vi "ReadMessage.vi"(0 "reference":refnum<class "VdTcpIP.lvclass">, 2 "MaxBytesToRead(10000)":u32=10000, 3 "Binary":bool, 4 "timeout ms (25000)":i32=25000, 5 "error in (no error)":errorcluster, 6 "mode (standard)":T1(ring)) -> (14 "reference out":refnum<class "VdTcpIP.lvclass">, 15 "Message":string, 19 "error out":errorcluster)   [LabVIEW 2020, in "VdTcpIP.lvclass"]
doc: "Reads a message"
uses:
  VdTcpIP.lvclass
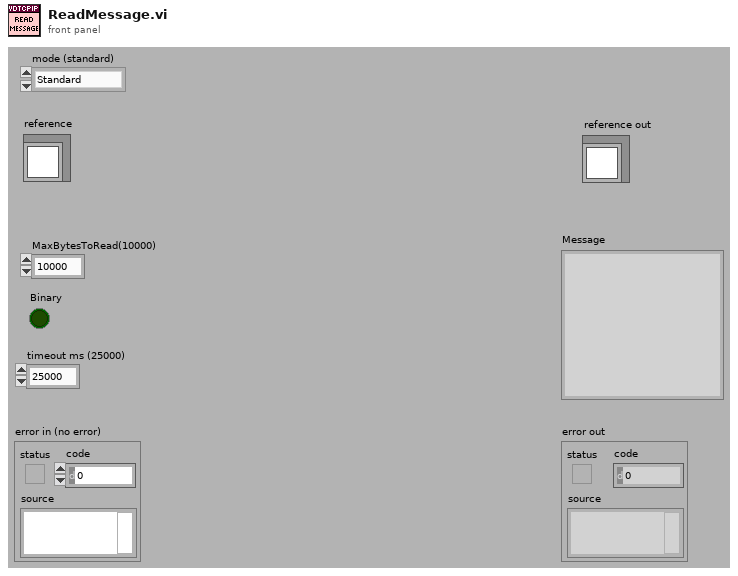
[diagram p1: front panel]
types:
  T1 = enum16{"Standard", "Buffered", "CRLF", "Immediate"}
  T2 = typedef "VdTcpIP.lvclass/ObjectAttributes.ctl" = cluster{"IP-Address":string, "Port":u16, "Connection":refnum<k5>, "Listener":refnum<k5>, "ListenerConnection":refnum<k5>, "Listner":bool, "ListnerProcessRunning":bool, "InConnections":refnum<k5>[], "InConnectionsIP":string[], "InConnectionAdded":refnum<notifier>, "RunVIOnNewConnection":variant, "DataToNewConnectionVI":cluster{"ControlName":string, "ControlValue":variant}[], "WebServicesURL_Location(http://...)":string, "WebServicesPostWebPage(*.asmx)":string, "Semaphore":T3, "AutoReConnectTimes":i32, "AutoReConnectInterval(ms)":i32, "ConnectionTimeout":i32}
  T3 = typedef "Semaphore RefNum" = refnum<k1>
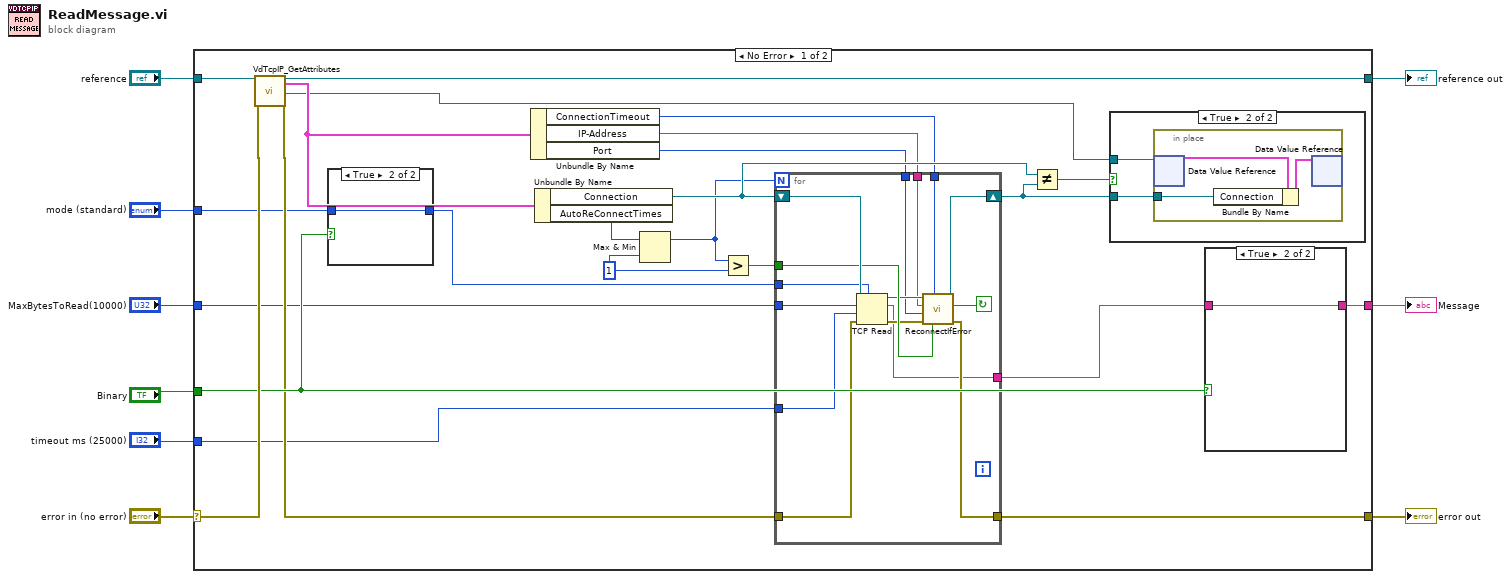
[diagram p0: block diagram]
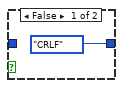
[diagram p3: hidden frame]
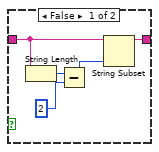
[diagram p4: hidden frame]
diagram:
  n1 = case shown="No Error" "error in (no error)" {
    selector: "error in (no error)" -> [w33 w62]
    tunnel: "reference" -> [w32 w63]
    tunnel: [w27 w62] -> w7
    tunnel: [w31 w63] -> w6
    tunnel: "timeout ms (25000)" -> [w23 _]
    tunnel: [w30 _] -> w4
    tunnel: "Binary" -> [w29 _]
    tunnel: "MaxBytesToRead(10000)" -> [w25 _]
    tunnel: "mode (standard)" -> [w10 _]
    frame No Error {
      w19 = 1 ("x")
      n2 = call "VdTcpIP_GetAttributes.vi"("reference in"=w32, "error in (no error)"=w33) -> ("reference out"=w31:refnum<class "VdTcpIP.lvclass">, "Data"=w21:T2, "DataRef"=w11:refnum<data-value>, "error out"=w28:errorcluster)  [unwired: 1 in, 13 out]
      n3 = case shown="True" w29 {
        tunnel: [T1."CRLF" ("mode (standard)") w55] -> w24
        tunnel: w10 -> [_ w55]
        frame False {
        }
        frame True {
        }
      }
      n4 = Unbundle By Name(w21) -> ("ConnectionTimeout"=w16:i32, "IP-Address"=w15:string, "Port"=w14:u16)
      n5 = Unbundle By Name(w21) -> ("Connection"=w22:refnum<k5>, "AutoReConnectTimes"=w20:i32)
      n6 = Max & Min(x=w20, y=w19) -> (max(x,y)=w18:i32)  [unwired: 1 out]
      n7 = Greater?(x=w18, y=w19) -> (0:w17:bool)
      n8 = for {
        N: w18 -> [_]
        tunnel: w23 -> [w51]
        tunnel: w17 -> [w50]
        tunnel: w28 -> [w53]
        tunnel: [w48] -> w27
        tunnel: w16 -> [w46]
        shift-right: [w44] -> w13
        shift-left: w22 -> [w52]
        tunnel: w15 -> [w43]
        tunnel: w14 -> [w42]
        tunnel: [w41] -> w26
        tunnel: w25 -> [w40]
        tunnel: w24 -> [w39]
        stop <- w47 continue-if-true
        n9 = TCP Read(connection ID=w52, bytes to read=w40, error in (no error)=w53, 7:w39, 9:w51) -> (connection ID out=w45:refnum<k5>, data out=w41:string, error out=w49:errorcluster)
        n10 = call "ReconnectIfError.vi"("TryReconnect"=w50, "ConnectionTimeout"=w46, "error in (no error)"=w49, "Port"=w42, "IP-Address"=w43, "TCP Network Connection in"=w45) -> ("error out"=w48:errorcluster, "TryAgain(Managed to Reconnect, and TryReconnect is True)"=w47:bool, "TCP Network Connection out"=w44:refnum<k5>)  [unwired: 3 in]
      }
      n11 = Not Equal?(x=w22, y=w13) -> (x != y?=w12:bool)
      n12 = case shown="True" w12 {
        tunnel: w11 -> [_ w35]
        tunnel: w13 -> [_ w34]
        frame False {
        }
        frame True {
          n13 = in-place {
            in-place-border: w34 -> [w36]
            n14 = in-place-dvr #1(w35) -> (w38:T2)  [unwired: 1 out]
            n15 = Bundle By Name(cluster=w38, "Connection"=w36) -> (w37:T2)
            n16 = in-place-dvr #1(w37) -> ()  [unwired: 2 out]
          }
        }
      }
      n17 = case shown="True" w29 {
        tunnel: w26 -> [w60 w61]
        tunnel: [w56 w61] -> w30
        frame False {
          n18 = String Length(string=w60) -> (length=w59:i32)
          n19 = Subtract(x=w59, y=2) -> (x-y=w57:i32)
          n20 = String Subset(string=w60, length (rest)=w57) -> (substring=w56:string)  [unwired: 1 out]
        }
        frame True {
        }
      }
    }
    frame Error {
    }
  }
  "reference out" <- w6
  "error out" <- w7
  "Message" <- w4
